vi "Configure RTD Type.vi"(8 "error in (no error)":errorcluster, 9 "Resistance at 0°C(100Ohm)":dbl=100.0, 10 "RTD Type":T1=enum."Pt3851" caption="RTD Type(Pt3851)", 11 "NI DMM Driver in":refnum<class "DMM.NI.lvclass">) -> (0 "error out":errorcluster, 1 "Success?":bool, 3 "NI DMM Driver out":refnum<class "DMM.NI.lvclass">)   [LabVIEW 2020, in "NI DMM Driver.lvlib" / "DMM.NI.lvclass"]
doc: "Configure the RTD type used when measuring temperatures."
uses:
  DMM.NI.lvclass
  PPL/HDH.Driver.DMM.lvlibp/Controls/Ctl_RTDType.ctl
  PPL/HDH.Driver.DMM.lvlibp
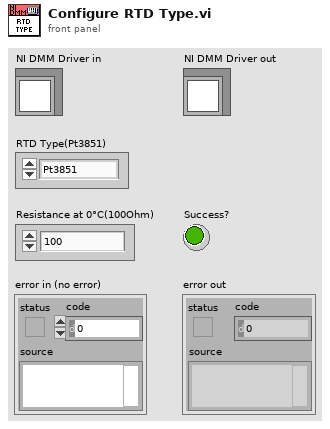
[diagram p1: front panel]
types:
  T1 = typedef "HDH.Driver.DMM.lvlibp/Ctl_RTDType.ctl" = enum16{"Custom", "Pt3750", "Pt3851", "Pt3911", "Pt3916", "Pt3920", "Pt3928"}
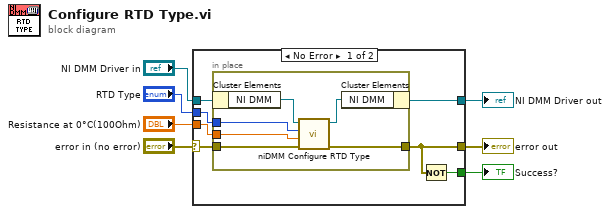
[diagram p0: block diagram]
diagram:
  n1 = case shown="No Error" "error in (no error)" {
    selector: "error in (no error)" -> [w10 w22]
    tunnel: [w9 w22] -> w6
    tunnel: [w13 w21] -> w5
    tunnel: "NI DMM Driver in" -> [w14 w21]
    tunnel: "RTD Type" -> [w12 _]
    tunnel: "Resistance at 0°C(100Ohm)" -> [w11 _]
    tunnel: [w8 _] -> w1
    frame No Error {
      n2 = in-place {
        in-place-border: w12 -> [w18]
        in-place-border: w11 -> [w17]
        in-place-border: w10 -> [w16]
        in-place-border: [w15] -> w9
        n3 = in-place-cluster #1(w14) -> ("NI DMM"=w20:refnum<k15>)
        n4 = call <instrlib>:"niDMM Configure RTD Type.vi"("error in (no error)"=w16, "RTD Resistance"=w17, "RTD Type"=w18, "instrument handle"=w20) -> ("error out"=w15:errorcluster, "instrument handle out"=w19:refnum<k15>)  [unwired: 6 in]
        n5 = in-place-cluster #1("NI DMM"=w19) -> (w13:refnum<class "DMM.NI.lvclass">)
      }
      n6 = Not(x=w9) -> (.not. x?=w8:bool)
    }
    frame Error {
    }
  }
  "error out" <- w6
  "NI DMM Driver out" <- w5
  "Success?" <- w1
